vi "Write Current_Share.vi"(8 "error in":errorcluster, 10 "Current_Sharing":bool, 11 "6700C in":refnum<class "6700C.lvclass">) -> (0 "error out":errorcluster, 3 "6700C out":refnum<class "6700C.lvclass">)   [LabVIEW 2019, in "6700C.lvlib" / "6700C.lvclass"]
uses:
  Library/6700C.lvclass
  builds/Instruments/PowerSupply.lvlibp/Library/PowerSupply.lvclass
  <vilib>/ErrorRing/Error Ring.xnode
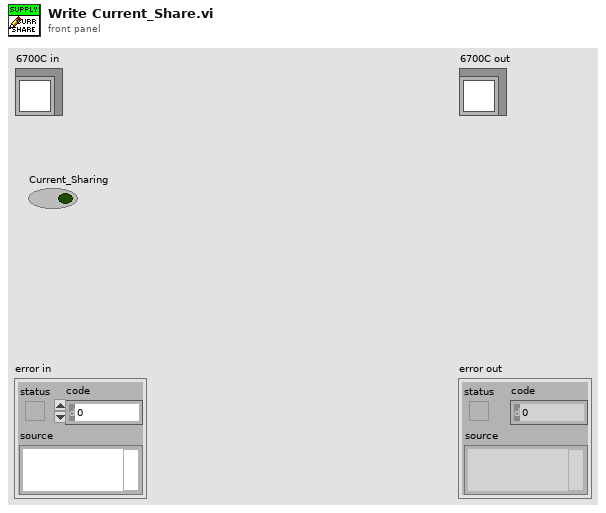
[diagram p1: front panel]
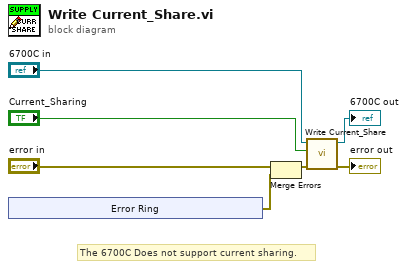
[diagram p0: block diagram]
diagram:
  # "The 6700C Does not support current sharing."
  n1 = xnode "Error Ring"() -> ("error out"=w3:errorcluster)
  n2 = Merge Errors("error in", w3) -> (w1:errorcluster)
  n3 = call-parent "Write Current_Share.vi"("error in"=w1, "Current_Sharing"="Current_Sharing", "PowerSupply in"="6700C in") -> ("error out"=→"error out":errorcluster, "PowerSupply out"=→"6700C out":refnum<class "6700C.lvclass">)  [unwired: 7 in]
